vi "W7X2DJSONwrong.vi"(4 "values":sgl[][](array[numeric]), 5 "label":string, 6 "dimensionSize":i32, 8 "dimensions":i64[](array[numeric]), 9 "dimensionCount":i32, 10 "sampleCount":i32, 11 "datatype":string) -> (3 "JSON string":string)   [LabVIEW 2014]
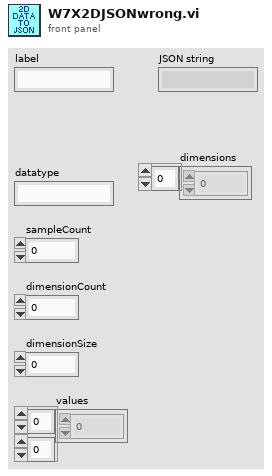
[diagram p1: front panel]
types:
  T1 = cluster{"label":string, "datatype":string, "sampleCount":i32, "dimensionCount":i32, "dimensionSize":i32, "values":sgl[][], "dimensions":i64[]}
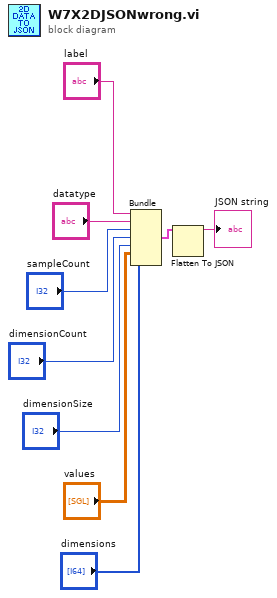
[diagram p0: block diagram]
diagram:
  n1 = Bundle("label"="label", "datatype"="datatype", "sampleCount"="sampleCount", "dimensionCount"="dimensionCount", "dimensionSize"="dimensionSize", "values"="values", "dimensions"="dimensions") -> (w5:T1)  [unwired: 1 in]
  n2 = Flatten To JSON(anything=w5) -> (JSON string=→"JSON string":string)  [unwired: 2 in, 1 out]
